vi "Init.vi"(8 "error in":errorcluster, 11 "object in":refnum<class "Scope PXI CFG.lvclass">) -> (0 "error out":errorcluster, 3 "object out":refnum<class "Scope PXI CFG.lvclass">)   [LabVIEW 2023, in "Scope.lvlib" / "Scope PXI.lvlib" / "Scope PXI CFG.lvclass"]
uses:
  Scope PXI CFG.lvclass
  Configuration Base/Configuration Base.lvclass/Configuration Base.ctl
  Scope PXI CFG.lvclass/Scope PXI CFG.ctl
  7f301f3d-d01a-4c51-ac1c-d6c990f17446.vi
  <vilib>/JDP Science/JSONtext/Find Item.vi
  <vilib>/JDP Science/JSONtext/Next JSON Value.vi
  <vilib>/JDP Science/JSONtext/String Subset.vi
  <vilib>/JDP Science/JSONtext/Parsing/Advance past next JSON Value (inlined COPY).vi
  <vilib>/JDP Science/JSONtext/Parsing/Advance past whitespace.vi
  <vilib>/JDP Science/JSONtext/Parsing/Advance past String.vi
  <vilib>/JDP Science/JSONtext/Parsing/Advance past Number.vi
  <vilib>/JDP Science/JSONtext/Parsing/Advance past Line Ending.vi
  <vilib>/JDP Science/JSONtext/Parsing/Parse Full Path or Item Name.vi
  <vilib>/JDP Science/JSONtext/Parsing/Advance past Array.vi
  <vilib>/JDP Science/JSONtext/Parsing/Advance past Object.vi
  <vilib>/JDP Science/JSONtext/support/Error Cluster From Code.vi
  <vilib>/JDP Science/JSONtext/Offset/Find Item Locations by Path.vi
  <vilib>/JDP Science/JSONtext/JSON text to Variant.vi
  <vilib>/Utility/error.llb/Error Cluster From Error Code.vi
  <vilib>/JDP Science/JSONtext/LVClass Serializer/JSONtext LVClass Serializer.lvclass
  <vilib>/ErrorRing/Error Ring.xnode
  Configuration Base/Configuration Base.lvclass
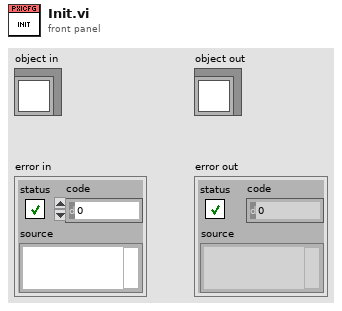
[diagram p1: front panel]
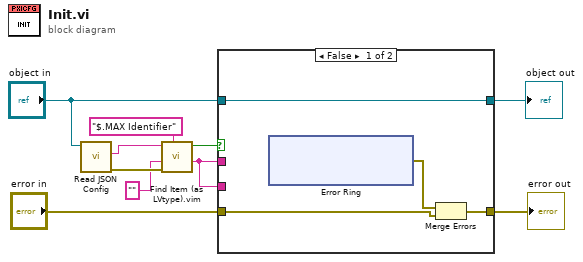
[diagram p0: block diagram]
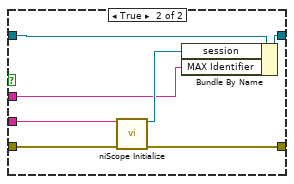
[diagram p2: hidden frame]
diagram:
  n1 = call "Read JSON Config.vi"("object in"="object in") -> ("error out"=w6:errorcluster, "<JSON>Config"=w7:string)  [unwired: 8 in, 1 out]
  n2 = call "Find Item (as LVtype).vim"("$Path or Item Name"="$.MAX Identifier", "error in (no error)"=w6, "Data Type and Default Value"="", "JSON"=w7) -> ("Data"=w2:string, "Found"=w1:bool)  [unwired: 4 in, 2 out]
  n3 = case shown="False" w1 {
    tunnel: "error in" -> [w12 w26]
    tunnel: [w14 w25] -> w9
    tunnel: [w11 w24] -> w8
    tunnel: "object in" -> [w11 w22]
    tunnel: w2 -> [_ w21]
    tunnel: w2 -> [_ w20]
    frame False {
      n4 = xnode "Error Ring"() -> ("error out"=w13:errorcluster)
      n5 = Merge Errors(w13, w12) -> (w14:errorcluster)
    }
    frame True {
      n6 = call <instrlib>:"niScope Initialize.vi"("resource name"=w21, "error in"=w26) -> ("instrument handle"=w23:refnum<k15>, "error out"=w25:errorcluster)  [unwired: 12 in]
      n7 = Bundle By Name(cluster=w22, "session"=w23, "MAX Identifier"=w20) -> (w24:refnum<class "Scope PXI CFG.lvclass">)
    }
  }
  "error out" <- w9
  "object out" <- w8
